vi "Fail Safe.vi"(10 "Value":bool, 11 "index":u16) -> (3 "function return":bool)   [LabVIEW 2025, in "ExtremelyEpicImagerIPC2.lvlib"]
doc: "IMAGERIPC_API bool WINAPI FailSafe(WORD index, bool Value);"
uses:
  ExtremelyEpicImagerIPC2.lvlib
  ImagerIPC2.dll
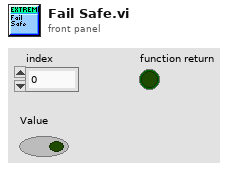
[diagram p1: front panel]
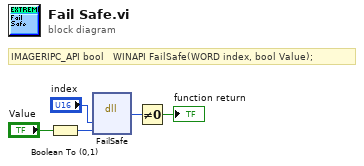
[diagram p0: block diagram]
diagram:
  # "IMAGERIPC_API bool   WINAPI FailSafe(WORD index, bool Value);"
  n1 = Boolean To (0,1)(Boolean="Value") -> (0, 1=w1:i16)
  n2 = dll-call lib="C:/Users/mayhe/OneDrive/Documents/GitHub/In-situ-monitoring-of-powder-bed-fusion-additive-manufacturing/system_development/Orichalcum/v0.2/Software_design/thermal-camera/VI/Connect SDK/ImagerIPC2.*" fn="FailSafe"("index"="index", "Value"=w1) -> (w4:u8)  [unwired: 5 in, 2 out]
  n3 = Not Equal To 0?(x=w4) -> (x != 0?=→"function return":bool)
